vi "toUNIX-Epoch.vi"(11 "Epoch in":refnum<class "Epoch.lvclass">) -> (2 "Unix Epoch Time":i64, 3 "Epoch":refnum<class "Epoch.lvclass">)   [LabVIEW 2013, in "Epoch.lvclass"]
uses:
  Epoch.lvclass
  Epoch.lvclass/Epoch.ctl
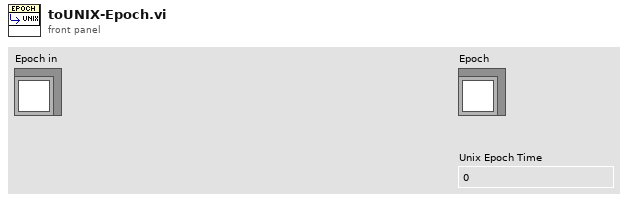
[diagram p1: front panel]
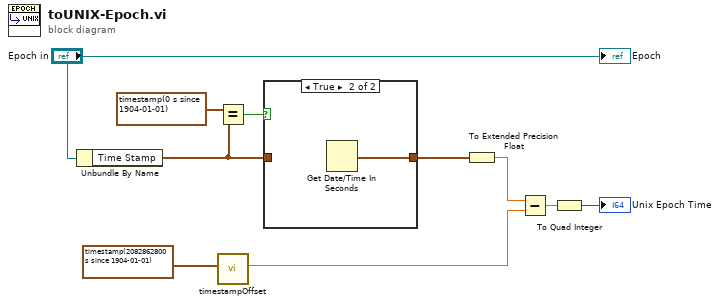
[diagram p0: block diagram]
diagram:
  n1 = Unbundle By Name("Epoch in") -> ("Time Stamp"=w7:timestamp)
  n2 = Equal?(x=timestamp(0 s since 1904-01-01), y=w7) -> (x = y?=w8:bool)
  n3 = call "timestampOffset.vi"("Reference Time"=timestamp(2082862800 s since 1904-01-01) ("current time")) -> ("Timestamp Offset"=w2:ext)  [unwired: 10 in]
  n4 = case shown="True" w8 {
    tunnel: [w11 w12] -> w5
    tunnel: w7 -> [w11 _]
    frame False {
    }
    frame True {
      n5 = Get Date/Time In Seconds() -> (seconds since 1Jan1904=w12:timestamp)
    }
  }
  n6 = To Extended Precision Float(1:w5) -> (0:w10:ext)
  n7 = Subtract(x=w10, y=w2) -> (x-y=w4:ext)
  n8 = To Quad Integer(1:w4) -> (0:→"Unix Epoch Time":i64)
  "Epoch" <- "Epoch in"
